vi "PhaseMapShift.vi"(8 "Phase scal":dbl, 9 "start":i32, 10 "V_y":dbl[](array[numeric]), 11 "Phase":dbl[](array[numeric])) -> (1 "Convert V to phase":dbl[](graph), 2 "Phase":dbl[][](graph))   [LabVIEW 2022 SP3]
uses:
  <vilib>/Analysis/NI_AALPro.lvlib
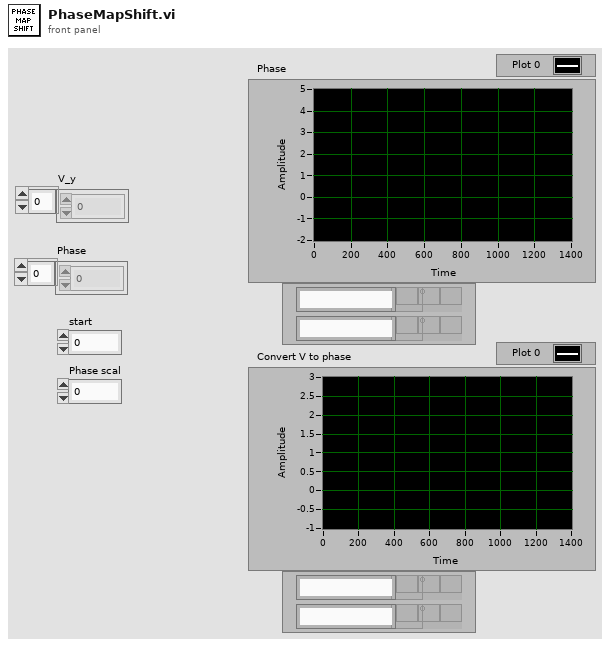
[diagram p1: front panel]
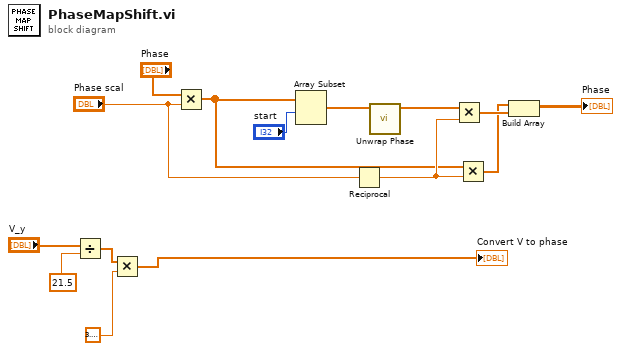
[diagram p0: block diagram]
diagram:
  n1 = Divide(x="V_y", y=21.5) -> (x/y=w3:dbl[])
  n2 = Multiply(x=w3, y=3.141592653589793) -> (x*y=→"Convert V to phase":dbl[])
  n3 = Multiply(x="Phase", y="Phase scal") -> (x*y=w7:dbl[])
  n4 = Array Subset(array=w7, index="start") -> (w8:dbl[])  [unwired: 1 in]
  n5 = Reciprocal(x="Phase scal") -> (1/x=w11:dbl)
  n6 = call <vilib>:"Unwrap Phase.vi"("Phase"=w8) -> ("Unwrapped Phase"=w13:dbl[])  [unwired: 9 in, 1 out]
  n7 = Multiply(x=w13, y=w11) -> (x*y=w10:dbl[])
  n8 = Multiply(x=w7, y=w11) -> (x*y=w9:dbl[])
  n9 = Build Array(w9, w10) -> (→"Phase":dbl[][])
